vi "Function_SaveCTRLparam.vi"(8 "error in (no error)":errorcluster, 9 "Class TCP":T1, 10 "Save CTRL params":bool, 11 "CS_IF_Params":T2 {"CS_Duty" min=0 max=1}) -> (0 "error out":errorcluster, 3 "Saved CTRL params ?":bool)   [LabVIEW 2021]
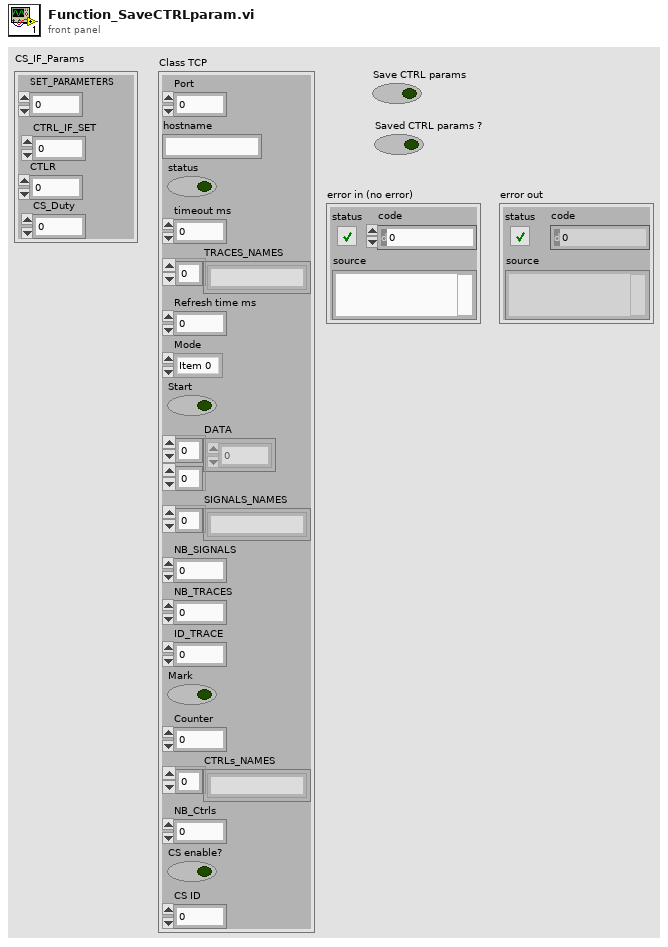
[diagram p1: front panel]
types:
  T1 = cluster{"Port":i32, "hostname":string, "status":bool, "timeout ms":i32, "TRACES_NAMES":string[], "Refresh time ms":i32, "Mode":enum32{"Item 0", "Item 1"}, "Start":bool, "DATA":sgl[][], "SIGNALS_NAMES":string[], "NB_SIGNALS":i32, "NB_TRACES":i32, "ID_TRACE":i32, "Mark":bool, "Counter":i32, "CTRLs_NAMES":string[], "NB_Ctrls":i32, "CS enable?":bool, "CS ID":i32}
  T2 = cluster{"SET_PARAMETERS":i32, "CTLR":i32, "CS_Duty":sgl, "CTRL_IF_SET":i32}
  T3 = cluster{"timeout ms":i32, "remote port":u16, "Address":string}
  T4 = cluster{"TRACE_SIZE":i32, "CS_ID":i32, "TRACE ID":i32, "CMD":i32, "DATA PARAM":string}
  T5 = enum16{"big-endian, network order", "native, host order", "little-endian"}
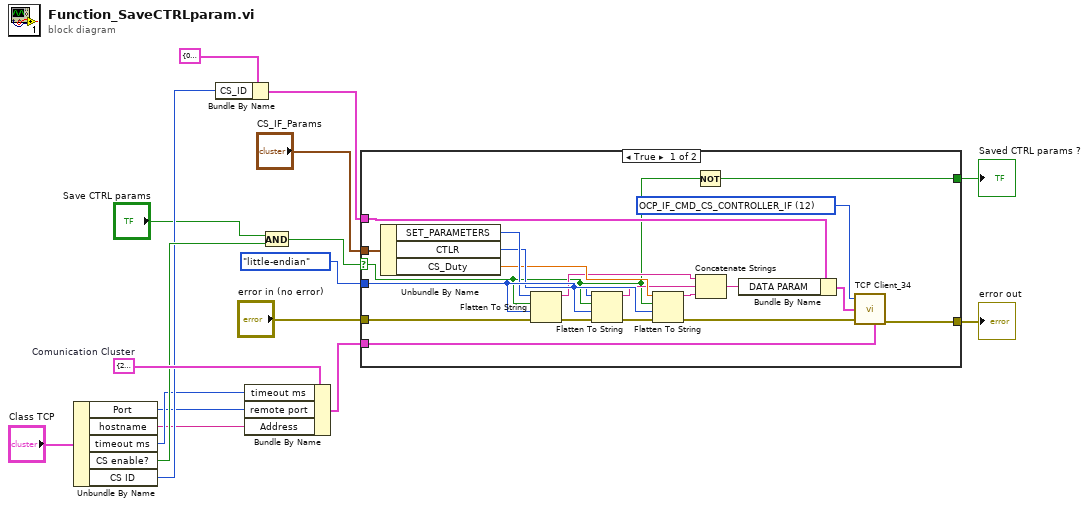
[diagram p0: block diagram]
diagram:
  w17 = T3 {"timeout ms"=2000, "remote port"=8085, "Address"="127.0.0.1"}  # Comunication Cluster
  n1 = Unbundle By Name("Class TCP") -> ("Port"=w5:i32, "hostname"=w6:string, "timeout ms"=w7:i32, "CS enable?"=w14:bool, "CS ID"=w13:i32)
  n2 = Bundle By Name(cluster=T4 {"TRACE_SIZE"=0, "CS_ID"=0, "TRACE ID"=0, "CMD"=0, "DATA PARAM"=""} ("Input Cluster"), "CS_ID"=w13) -> (w12:T4)
  n3 = Bundle By Name(cluster=w17, "timeout ms"=w7, "remote port"=w5, "Address"=w6) -> (w8:T3)
  n4 = And(x="Save CTRL params", y=w14) -> (x .and. y?=w4:bool)
  n5 = case shown="True" w4 {
    selector: w4 -> [w20 w38]
    tunnel: w8 -> [w37 _]
    tunnel: "error in (no error)" -> [w35 w39]
    tunnel: w12 -> [w36 _]
    tunnel: [w34 w39] -> w9
    tunnel: "CS_IF_Params" -> [w33 _]
    tunnel: T5."little-endian" ("byte order (0:big-endian, network order)") -> [w32 _]
    tunnel: [w19 w38] -> w15
    frame True {
      w31 = 12 items=["OCP_IF_CMD_TRACE_READ", "OCP_IF_CMD_TRACE_RESET", "OCP_IF_CMD_TRACE_GET_SIZE", "OCP_IF_CMD_TRACE_SET_SIZE", "OCP_IF_CMD_TRACE_GET_NUMBER_SIGNALS", "OCP_IF_CMD_TRACE_GET_SIGNALS_NAMES", "OCP_IF_CMD_TRACE_GET_NUMBER_TRACES", "OCP_IF_CMD_TRACE_GET_TRACES_NAMES", "OCP_IF_CMD_TRACE_GET_ADDRESS", "OCP_IF_CMD_CS_STATUS", "OCP_IF_CMD_CS_ENABLE", "OCP_IF_CMD_CS_DISABLE", "OCP_IF_CMD_CS_CONTROLLER_IF", "OCP_IF_CMD_CS_HARDWARE_IF", "OCP_IF_CMD_CS_GET_NUMBER_CONTROLLERS", "OCP_IF_CMD_CS_GET_CONTROLLERS_NAMES", "OCP_IF_CMD_PLATFORM_ID", "OCP_IF_CMD_PLATFORM_IF", "OCP_IF_CMD_OPIL_UPDATE_MEASUREMENTS", "OCP_IF_CMD_OPIL_UPDATE_SIM_DATA", "OCP_IF_CMD_OPIL_RUN_CONTROL", "OCP_IF_CMD_OPIL_INITIALIZE_CONTROL", "OCP_IF_CMD_OPIL_GET_CONTROL", "OCP_IF_CMD_OPIL_GET_CONTROLLER_DATA", "OCP_IF_CMD_END"] ("CMD")
      n6 = Unbundle By Name(w33) -> ("SET_PARAMETERS"=w28:i32, "CTLR"=w27:i32, "CS_Duty"=w26:sgl)
      n7 = Flatten To String(anything=w28, prepend array or string size? (T)=w20, byte order (0:big-endian, network order)=w32, error in (no error)=w35) -> (data string=w25:string, error out=w30:errorcluster)  [unwired: 1 out]
      n8 = Flatten To String(anything=w27, prepend array or string size? (T)=w20, byte order (0:big-endian, network order)=w32, error in (no error)=w30) -> (data string=w24:string, error out=w29:errorcluster)  [unwired: 1 out]
      n9 = Flatten To String(anything=w26, prepend array or string size? (T)=w20, byte order (0:big-endian, network order)=w32, error in (no error)=w29) -> (data string=w23:string, error out=w18:errorcluster)  [unwired: 1 out]
      n10 = Not(x=w20) -> (.not. x?=w19:bool)
      n11 = Concatenate Strings(w25, w24, w23) -> (w21:string)
      n12 = Bundle By Name(cluster=w36, "DATA PARAM"=w21) -> (w22:T4)
      n13 = call "TCP Client_34.vi"("CMD"=w31, "Input Cluster"=w22, "error in (no error)"=w18, "Comunication Cluster"=w37) -> ("error out"=w34:errorcluster)  [unwired: 4 in, 2 out]
    }
    frame False {
    }
  }
  "Saved CTRL params ?" <- w15
  "error out" <- w9
